vi "Main.vi"() -> ()   [LabVIEW 2013]
uses:
  <vilib>/Utility/error.llb/DialogType.ctl
panel:
  out "error out":errorcluster
  out "Pomiary":dbl[](array[numeric])
  in  "stop":bool
  out "Waveform Chart":dbl(graph)
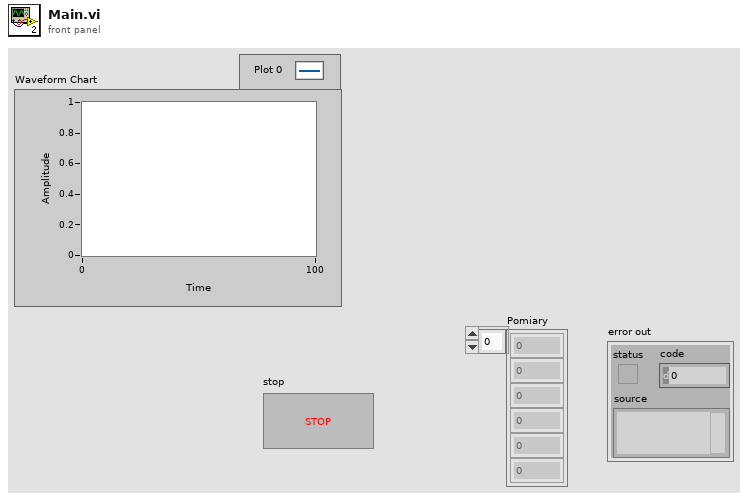
[diagram p1: front panel]
types:
  T1 = typedef "DialogType.ctl" = u16
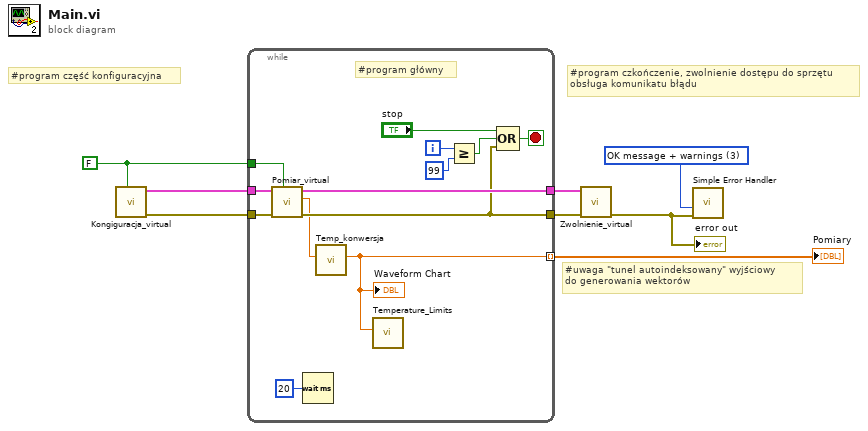
[diagram p0: block diagram]
diagram:
  w6 = FALSE ("Error Generate")
  w8 = T1 3 items=["no dialog", "OK message", "continue or stop message", "OK message + warnings", "continue/stop + warnings"] ("type of dialog (OK msg:1)")
  # "#program część konfiguracyjna"
  # "#program czkończenie, zwolnienie dostępu do sprzętu\nobsługa komunikatu błądu"
  # "#uwaga \"tunel autoindeksowany\" wyjściowy\ndo generowania wektorów"
  n1 = call "Kongiguracja_virtual.vi"("Error Generate"=w6) -> ("error out"=w1:errorcluster, "Reference out"=w2:cluster{"Numeric":dbl, "Boolean":bool})  [unwired: 9 in]
  n2 = while {
    tunnel: w1 -> [w16]
    tunnel: [w11] -> w5
    tunnel: [w14] -> w3
    tunnel: [w10] -> w7 mode=indexing
    tunnel: w2 -> [w15]
    tunnel: w6 -> [w13]
    i -> [w18]
    stop <- w19 stop-if-true
    # "#program główny"
    n3 = call "Pomiar_virtual.vi"("Error Generate"=w13, "error in (no error)"=w16, "Reference in"=w15) -> ("error out"=w11:errorcluster, "out"=w9:dbl, "Reference out"=w14:cluster{"Numeric":dbl, "Boolean":bool})  [unwired: 6 in]
    n4 = Wait (ms)(milliseconds to wait=u32 20) -> ()  [unwired: 1 out]
    n5 = call "Temp_konwersja.vi"("Temp in"=w9) -> ("Temp out"=w10:dbl)  [unwired: 9 in, 1 out]
    "Waveform Chart" <- w10
    n6 = call "Temperature_Limits.vi"("TEMP"=w10) -> ()  [unwired: 8 in, 3 out]
    n7 = Greater Or Equal?(x=w18, y=99) -> (x >= y?=w12:bool)
    n8 = Compound Arithmetic op=OR("stop", w12, w11) -> (w19:bool)
  }
  "Pomiary" <- w7
  n9 = call "Zwolnienie_virtual.vi"("error in (no error)"=w5, "Reference in"=w3) -> ("error out"=w4:errorcluster)  [unwired: 9 in]
  "error out" <- w4
  n10 = call <vilib>:"Simple Error Handler.vi"("type of dialog (OK msg:1)"=w8, "error in (no error)"=w4) -> ()  [unwired: 3 in, 5 out]
